vi "NUMtoSTRING.vi"(11 "number":i32) -> (3 "decimal integer string":string)   [LabVIEW 2016]
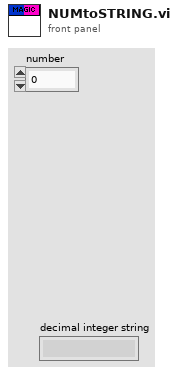
[diagram p1: front panel]
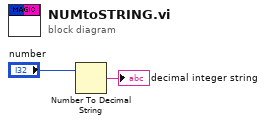
[diagram p0: block diagram]
diagram:
  n1 = Number To Decimal String(number="number") -> (decimal integer string=→"decimal integer string":string)  [unwired: 1 in]
